vi "fgv_pid-config.vi"(7 "cmd":enum16{"read", "write"}(ring), 8 "error in":errorcluster, 11 "PID cfg":T1={"PID gains"={"proportional gain (Kc)"=0.002499999999999999, "integral time (Ti, min)"=0.0, "derivative time (Td, min)"=0.0}, "PID limits"={"output high"=0.07, "output low"=-0.07}, "dt_pid"=100} {"PID limits"."output low" format="%.3f"; "PID limits"."output high" format="%.3f"; "PID gains"."derivative time (Td, min)" format="%.4f"; "PID gains"."integral time (Ti, min)" format="%.4f"; "PID gains"."proportional gain (Kc)" format="%.4f"}) -> (0 "error out":errorcluster, 3 "PID cfg out":T1={"PID gains"={"proportional gain (Kc)"=0.002499999999999999, "integral time (Ti, min)"=0.0, "derivative time (Td, min)"=0.0}, "PID limits"={"output high"=0.07, "output low"=-0.07}, "dt_pid"=100} {"PID limits"."output low" format="%.3f"; "PID limits"."output high" format="%.3f"; "PID gains"."derivative time (Td, min)" format="%.4f"; "PID gains"."integral time (Ti, min)" format="%.4f"; "PID gains"."proportional gain (Kc)" format="%.4f"})   [LabVIEW 2019]
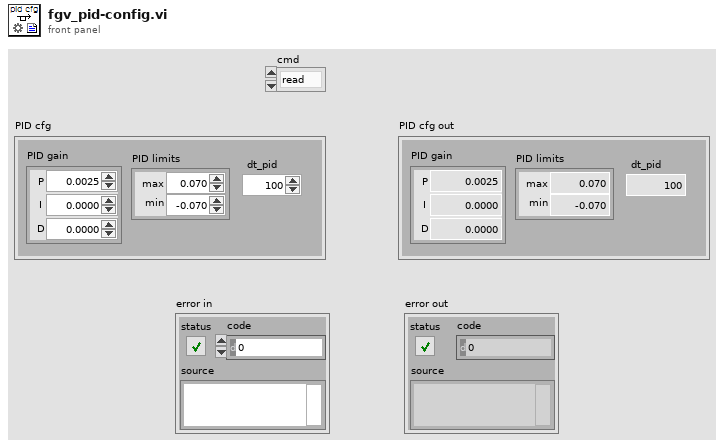
[diagram p1: front panel]
types:
  T1 = cluster{"PID gains":cluster{"proportional gain (Kc)":dbl, "integral time (Ti, min)":dbl, "derivative time (Td, min)":dbl}, "PID limits":cluster{"output high":dbl, "output low":dbl}, "dt_pid":u32}
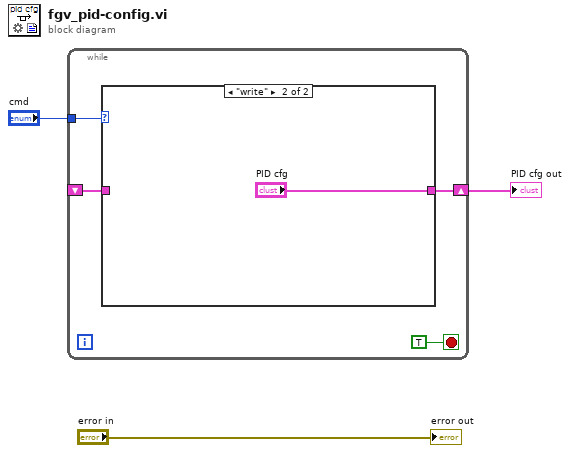
[diagram p0: block diagram]
diagram:
  n1 = while {
    shift-right: [w6] -> w1
    shift-left: _ -> [w5]
    tunnel: "cmd" -> [w4]
    stop <- TRUE stop-if-true
    n2 = case shown="\"write\"" w4 {
      tunnel: [w8 "PID cfg"] -> w6
      tunnel: w5 -> [w8 _]
      frame "read", Default {
      }
      frame "write" {
      }
    }
  }
  "PID cfg out" <- w1
  "error out" <- "error in"
